vi "file_readWriteState.vi"(7 "error in (no error)":errorcluster, 9 "file RefNum":refnum<file>) -> (0 "error out":errorcluster, 2 "access (0:read/write)":enum16{"read/write", "read-only", "write-only"}(ring))   [LabVIEW 2010]
panel:
  in  "file path (use dialog)":path
  out "data string":string
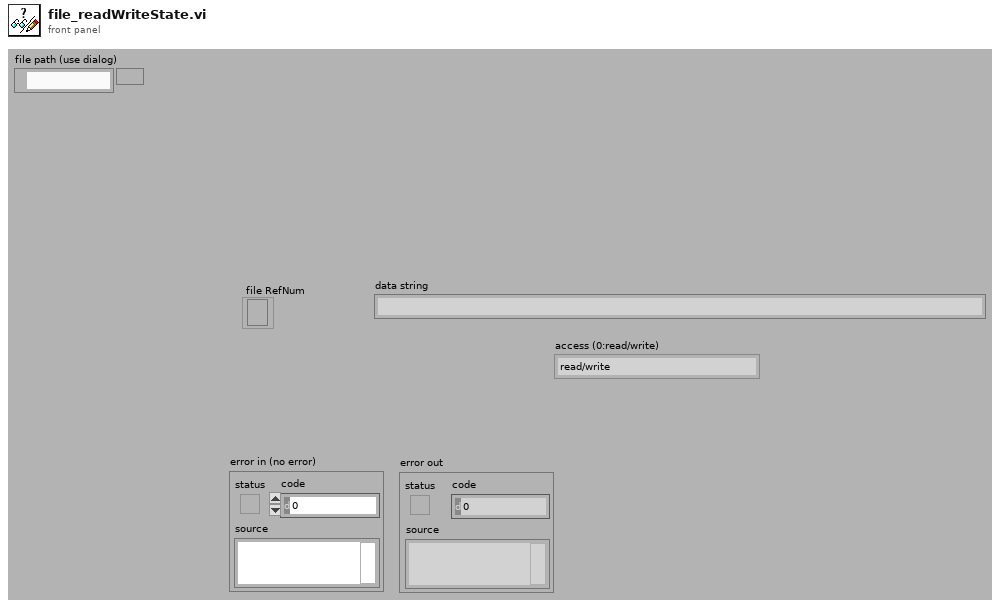
[diagram p1: front panel]
types:
  T1 = enum16{"open", "replace", "create", "open or create", "replace or create", "replace or create with confirmation"}
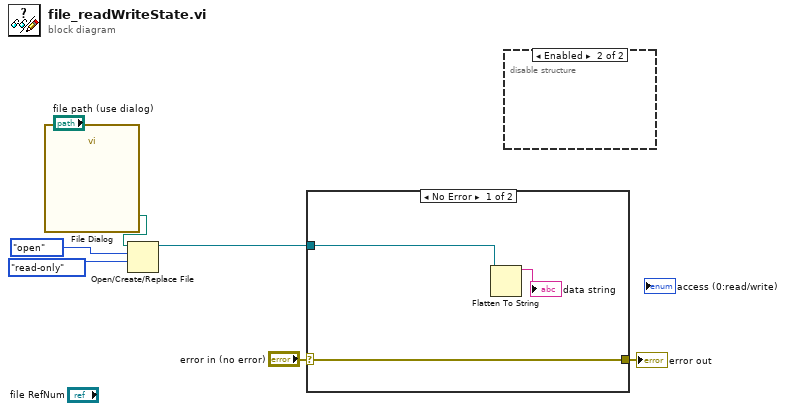
[diagram p0: block diagram]
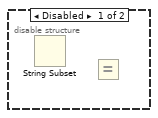
[diagram p3: hidden frame]
diagram:
  n1 = call "File Dialog"() -> ("selected path"=w4:path)  [unwired: 12 in, 3 out]
  n2 = Open/Create/Replace File(file path (use dialog)=w4, operation (0:open)=T1."open", access (0:read/write)=enum16{"read/write", "read-only", "write-only"}."read-only" ("access (0:read/write) 2")) -> (refnum out=w2:refnum<file>)  [unwired: 3 in, 2 out]
  n3 = case shown="No Error" "error in (no error)" {
    selector: "error in (no error)" -> [w8 w10]
    tunnel: w2 -> [w9 _]
    tunnel: [w8 w10] -> w1
    frame No Error {
      n4 = Flatten To String(anything=w9) -> (data string=→"data string":string)  [unwired: 3 in, 2 out]
    }
    frame Error {
    }
  }
  "error out" <- w1
  n5 = disable-structure shown="Enabled" {
    frame Disabled {
      n6 = String Subset() -> ()  [unwired: 3 in, 1 out]
      n7 = Equal?() -> ()  [unwired: 2 in, 1 out]
    }
    frame Enabled {
    }
  }
